vi "诊断标定3 - 副本.vi"(8 "CAN端口":u16(ring), 9 "设备索引号":u16(ring), 10 "CAN卡类型":u32(ring)=21) -> ()   [LabVIEW 2013] (continued)
            n1286 = Select(t=0, s=w1771, f=1) -> (s? t:f=w1770:i32)
            n1287 = property on="电池实际容量(A)" class="DigNum (严格)"("Disabled"=w1770) -> ()  [unwired: 2 in, 2 out]
            n1288 = property on="电池额定容量(A)" class="DigNum (严格)"("Disabled"=w1770) -> ()  [unwired: 2 in, 2 out]
            n1289 = property on="项目信息2" class="Clust (严格)"("DisabledEnum"=w1770) -> ()  [unwired: 2 in, 2 out]
            n1290 = global read "功能码全局.vi" "主板项目信息7"() -> (w1777:bool[])
            n1291 = Index Array(array=w1777, index #1=3 ("索引"), index #2=6 ("索引")) -> (element #1=w1775:bool, element #2=w1774:bool)
            n1292 = Not(x=w1781) -> (.not. x?=w1780:bool)
          }
          frame "配置文件版本" {
            w1794 = 2
            w1796 = FALSE
            n1293 = property on="使用者" class="DigNum (严格)"("Disabled"=w1794) -> ()  [unwired: 2 in, 2 out]
            n1294 = property on="SOH(%)" class="DigNum (严格)"("Disabled"=w1794) -> ()  [unwired: 2 in, 2 out]
            n1295 = property on="SOC(%)" class="DigNum (严格)"("Disabled"=w1794) -> ()  [unwired: 2 in, 2 out]
            n1296 = property on="电池实际容量(A)" class="DigNum (严格)"("Disabled"=w1794) -> ()  [unwired: 2 in, 2 out]
            n1297 = property on="从板个数" class="DigNum (严格)"("NumText.BGColor"=u32 13816530) -> ()  [unwired: 2 in, 2 out]
            n1298 = property on="电池额定容量(A)" class="DigNum (严格)"("Disabled"=w1794) -> ()  [unwired: 2 in, 2 out]
            n1299 = property on="系统时钟" class="Str"("Disabled"=w1794) -> ()  [unwired: 2 in, 2 out]
            n1300 = property on="车架(牌)号" class="Str"("Disabled"=w1794) -> ()  [unwired: 2 in, 2 out]
            n1301 = property on="项目信息" class="Tbl (严格)"("Disabled"=w1794) -> ()  [unwired: 2 in, 2 out]
            n1302 = property on="产品编号" class="Str"("Disabled"=w1794) -> ()  [unwired: 2 in, 2 out]
            n1303 = Select(t=0, s=w1785, f=1) -> (s? t:f=w1784:i32)
            n1304 = property on="项目信息2" class="Clust (严格)"("DisabledEnum"=w1784) -> ()  [unwired: 2 in, 2 out]
            n1305 = property on="配置文件版本" class="Str"("Disabled"=w1784) -> ()  [unwired: 2 in, 2 out]
            n1306 = global read "功能码全局.vi" "主板项目信息5"() -> (w1792:bool[])
            n1307 = global read "功能码全局.vi" "主板项目信息6"() -> (w1791:bool[])
            n1308 = Index Array(array=w1792, index=6 ("索引")) -> (element=w1789:bool)
            n1309 = Index Array(array=w1791, index=7 ("索引")) -> (element=w1788:bool)
            n1310 = Not(x=w1796) -> (.not. x?=w1795:bool)
          }
          frame "参数修改记录" {
            w1809 = 2
            w1811 = FALSE
            n1311 = property on="SOH(%)" class="DigNum (严格)"("Disabled"=w1809) -> ()  [unwired: 2 in, 2 out]
            n1312 = property on="SOC(%)" class="DigNum (严格)"("Disabled"=w1809) -> ()  [unwired: 2 in, 2 out]
            n1313 = property on="电池实际容量(A)" class="DigNum (严格)"("Disabled"=w1809) -> ()  [unwired: 2 in, 2 out]
            n1314 = property on="电池额定容量(A)" class="DigNum (严格)"("Disabled"=w1809) -> ()  [unwired: 2 in, 2 out]
            n1315 = property on="从板个数" class="DigNum (严格)"("NumText.BGColor"=u32 13816530) -> ()  [unwired: 2 in, 2 out]
            n1316 = property on="系统时钟" class="Str"("Disabled"=w1809) -> ()  [unwired: 2 in, 2 out]
            n1317 = property on="车架(牌)号" class="Str"("Disabled"=w1809) -> ()  [unwired: 2 in, 2 out]
            n1318 = property on="配置文件版本" class="Str"("Disabled"=w1809) -> ()  [unwired: 2 in, 2 out]
            n1319 = property on="项目信息" class="Tbl (严格)"("Disabled"=w1809) -> ()  [unwired: 2 in, 2 out]
            n1320 = property on="产品编号" class="Str"("Disabled"=w1809) -> ()  [unwired: 2 in, 2 out]
            n1321 = Select(t=0, s=w1800, f=1) -> (s? t:f=w1799:i32)
            n1322 = property on="使用者" class="DigNum (严格)"("Disabled"=w1799) -> ()  [unwired: 2 in, 2 out]
            n1323 = property on="项目信息2" class="Clust (严格)"("DisabledEnum"=w1799) -> ()  [unwired: 2 in, 2 out]
            n1324 = global read "功能码全局.vi" "主板项目信息7"() -> (w1806:bool[])
            n1325 = global read "功能码全局.vi" "主板项目信息5"() -> (w1807:bool[])
            n1326 = Index Array(array=w1806, index=0 ("索引")) -> (element=w1804:bool)
            n1327 = Index Array(array=w1807, index=7 ("索引")) -> (element=w1803:bool)
            n1328 = Not(x=w1811) -> (.not. x?=w1810:bool)
          }
          frame "车牌号" {
            w1824 = 2
            w1826 = FALSE
            n1329 = property on="SOH(%)" class="DigNum (严格)"("Disabled"=w1824) -> ()  [unwired: 2 in, 2 out]
            n1330 = property on="使用者" class="DigNum (严格)"("Disabled"=w1824) -> ()  [unwired: 2 in, 2 out]
            n1331 = property on="SOC(%)" class="DigNum (严格)"("Disabled"=w1824) -> ()  [unwired: 2 in, 2 out]
            n1332 = property on="电池实际容量(A)" class="DigNum (严格)"("Disabled"=w1824) -> ()  [unwired: 2 in, 2 out]
            n1333 = property on="电池额定容量(A)" class="DigNum (严格)"("Disabled"=w1824) -> ()  [unwired: 2 in, 2 out]
            n1334 = property on="从板个数" class="DigNum (严格)"("NumText.BGColor"=u32 13816530) -> ()  [unwired: 2 in, 2 out]
            n1335 = property on="系统时钟" class="Str"("Disabled"=w1824) -> ()  [unwired: 2 in, 2 out]
            n1336 = property on="配置文件版本" class="Str"("Disabled"=w1824) -> ()  [unwired: 2 in, 2 out]
            n1337 = property on="项目信息" class="Tbl (严格)"("Disabled"=w1824) -> ()  [unwired: 2 in, 2 out]
            n1338 = property on="产品编号" class="Str"("Disabled"=w1824) -> ()  [unwired: 2 in, 2 out]
            n1339 = Select(t=0, s=w1815, f=1) -> (s? t:f=w1814:i32)
            n1340 = property on="车架(牌)号" class="Str"("Disabled"=w1814) -> ()  [unwired: 2 in, 2 out]
            n1341 = property on="项目信息2" class="Clust (严格)"("DisabledEnum"=w1814) -> ()  [unwired: 2 in, 2 out]
            n1342 = global read "功能码全局.vi" "主板项目信息7"() -> (w1821:bool[])
            n1343 = global read "功能码全局.vi" "主板项目信息6"() -> (w1822:bool[])
            n1344 = Index Array(array=w1821, index=1 ("索引")) -> (element=w1819:bool)
            n1345 = Index Array(array=w1822, index=0 ("索引")) -> (element=w1818:bool)
            n1346 = Not(x=w1826) -> (.not. x?=w1825:bool)
          }
          frame "SOH" {
            w1838 = 2
            w1840 = FALSE
            n1347 = property on="使用者" class="DigNum (严格)"("Disabled"=w1838) -> ()  [unwired: 2 in, 2 out]
            n1348 = property on="SOC(%)" class="DigNum (严格)"("Disabled"=w1838) -> ()  [unwired: 2 in, 2 out]
            n1349 = property on="电池实际容量(A)" class="DigNum (严格)"("Disabled"=w1838) -> ()  [unwired: 2 in, 2 out]
            n1350 = property on="电池额定容量(A)" class="DigNum (严格)"("Disabled"=w1838) -> ()  [unwired: 2 in, 2 out]
            n1351 = property on="从板个数" class="DigNum (严格)"("NumText.BGColor"=u32 13816530) -> ()  [unwired: 2 in, 2 out]
            n1352 = property on="系统时钟" class="Str"("Disabled"=w1838) -> ()  [unwired: 2 in, 2 out]
            n1353 = property on="配置文件版本" class="Str"("Disabled"=w1838) -> ()  [unwired: 2 in, 2 out]
            n1354 = property on="项目信息" class="Tbl (严格)"("Disabled"=w1838) -> ()  [unwired: 2 in, 2 out]
            n1355 = property on="产品编号" class="Str"("Disabled"=w1838) -> ()  [unwired: 2 in, 2 out]
            n1356 = property on="车架(牌)号" class="Str"("Disabled"=w1838) -> ()  [unwired: 2 in, 2 out]
            n1357 = Select(t=0, s=w1830, f=1) -> (s? t:f=w1829:i32)
            n1358 = property on="项目信息2" class="Clust (严格)"("DisabledEnum"=w1829) -> ()  [unwired: 2 in, 2 out]
            n1359 = property on="SOH(%)" class="DigNum (严格)"("Disabled"=w1829) -> ()  [unwired: 2 in, 2 out]
            n1360 = global read "功能码全局.vi" "主板项目信息7"() -> (w1837:bool[])
            n1361 = Index Array(array=w1837, index #1=4 ("索引"), index #2=7 ("索引")) -> (element #1=w1834:bool, element #2=w1833:bool)
            n1362 = Not(x=w1840) -> (.not. x?=w1839:bool)
          }
          frame "SOC过低(2)", "SOC过高(2)", "SOH过低(2)", "充电电流过高(2)", "单体电压过低(2)", "单体电压过高(2)", "单组电压不均衡(2)", "单组温度不均衡(2)", "二级故障阀值", "放电电流过高(2)", "极柱温度过高(2)", "内阻过大(2)", "温度过低(2)", "温度过高(2)", "整组电压不均衡(2)", "整组温度不均衡(2)", "总电压过低(2)", "总电压过高(2)" {
            w1852 = FALSE
            n1363 = property on="从板个数" class="DigNum (严格)"("NumText.BGColor"=u32 13816530) -> ()  [unwired: 2 in, 2 out]
            n1364 = Select(t=0, s=w1844, f=1) -> (s? t:f=w1843:i32)
            n1365 = property on="一级故障 2" class="Clust (严格)"("DisabledEnum"=w1843) -> ()  [unwired: 2 in, 2 out]
            n1366 = global read "功能码全局.vi" "主板故障阀值9"() -> (w1850:bool[])
            n1367 = Index Array(array=w1850, index #1=3 ("索引"), index #2=6 ("索引")) -> (element #1=w1848:bool, element #2=w1847:bool)
            n1368 = Not(x=w1852) -> (.not. x?=w1853:bool)
          }
          frame "SOC过低(3)", "SOC过高(3)", "SOH过低(3)", "充电电流过高(3)", "单体电压过低(3)", "单体电压过高(3)", "单组电压不均衡(3)", "单组温度不均衡(3)", "放电电流过高(3)", "极柱温度过高(3)", "内阻过大(3)", "三级故障阀值", "温度过低(3)", "温度过高(3)", "整组电压不均衡(3)", "整组温度不均衡(3)", "总电压过低(3)", "总电压过高(3)" {
            w1866 = FALSE
            n1369 = property on="从板个数" class="DigNum (严格)"("NumText.BGColor"=u32 13816530) -> ()  [unwired: 2 in, 2 out]
            n1370 = Select(t=0, s=w1857, f=1) -> (s? t:f=w1856:i32)
            n1371 = property on="一级故障 3" class="Clust (严格)"("DisabledEnum"=w1856) -> ()  [unwired: 2 in, 2 out]
            n1372 = global read "功能码全局.vi" "主板故障阀值9"() -> (w1863:bool[])
            n1373 = Index Array(array=w1863, index #1=4 ("索引"), index #2=7 ("索引")) -> (element #1=w1861:bool, element #2=w1860:bool)
            n1374 = Not(x=w1866) -> (.not. x?=w1865:bool)
          }
          frame "SOC过低", "SOC过高", "SOH过低", "充电电流过高", "单体电压过低", "单体电压过高", "单组电压不均衡", "单组温度不均衡", "放电电流过高", "极柱温度过高", "内阻过大", "温度过低", "温度过高", "一级故障阀值", "整组电压不均衡", "整组温度不均衡", "总电压过低", "总电压过高" {
            w1879 = FALSE
            n1375 = Select(t=0, s=w1870, f=1) -> (s? t:f=w1869:i32)
            n1376 = property on="从板个数" class="DigNum (严格)"("NumText.BGColor"=u32 13816530) -> ()  [unwired: 2 in, 2 out]
            n1377 = property on="一级故障" class="Clust (严格)"("DisabledEnum"=w1869) -> ()  [unwired: 2 in, 2 out]
            n1378 = global read "功能码全局.vi" "主板故障阀值9"() -> (w1876:bool[])
            n1379 = Index Array(array=w1876, index #1=2 ("索引"), index #2=5 ("索引")) -> (element #1=w1874:bool, element #2=w1873:bool)
            n1380 = Not(x=w1879) -> (.not. x?=w1878:bool)
          }
          frame "充电控制参数", "电流步长", "最大允许充电电流", "最大允许充电温度", "最大允许单体电压", "最大允许总电压", "最小允许充电电流", "最小允许充电温度", "最小允许单体电压" {
            w1882 = 2
            w1893 = FALSE
            n1381 = property on="从板个数" class="DigNum (严格)"("NumText.BGColor"=u32 13816530) -> ()  [unwired: 2 in, 2 out]
            n1382 = property on="风机开启温度" class="DigNum (严格)"("Disabled"=w1882) -> ()  [unwired: 2 in, 2 out]
            n1383 = property on="风机关闭温度" class="DigNum (严格)"("Disabled"=w1882) -> ()  [unwired: 2 in, 2 out]
            n1384 = property on="加热开启温度" class="DigNum (严格)"("Disabled"=w1882) -> ()  [unwired: 2 in, 2 out]
            n1385 = property on="加热关闭温度" class="DigNum (严格)"("Disabled"=w1882) -> ()  [unwired: 2 in, 2 out]
            n1386 = property on="风机开启温差" class="DigNum (严格)"("Disabled"=w1882) -> ()  [unwired: 2 in, 2 out]
            n1387 = property on="风机关闭温差" class="DigNum (严格)"("Disabled"=w1882) -> ()  [unwired: 2 in, 2 out]
            n1388 = property on="加热控制参数" class="Clust (严格)"("DisabledEnum"=w1882) -> ()  [unwired: 2 in, 2 out]
            n1389 = Select(t=0, s=w1884, f=1) -> (s? t:f=w1883:i32)
            n1390 = property on="最大允许总电压" class="DigNum (严格)"("Disabled"=w1883) -> ()  [unwired: 2 in, 2 out]
            n1391 = property on="最大允许充电温度" class="DigNum (严格)"("Disabled"=w1883) -> ()  [unwired: 2 in, 2 out]
            n1392 = property on="最小允许充电温度" class="DigNum (严格)"("Disabled"=w1883) -> ()  [unwired: 2 in, 2 out]
            n1393 = property on="电流步长" class="DigNum (严格)"("Disabled"=w1883) -> ()  [unwired: 2 in, 2 out]
            n1394 = property on="最大允许单体电压" class="DigNum (严格)"("Disabled"=w1883) -> ()  [unwired: 2 in, 2 out]
            n1395 = property on="最小允许单体电压" class="DigNum (严格)"("Disabled"=w1883) -> ()  [unwired: 2 in, 2 out]
            n1396 = property on="最大允许充电电流" class="DigNum (严格)"("Disabled"=w1883) -> ()  [unwired: 2 in, 2 out]
            n1397 = property on="最小允许充电电流" class="DigNum (严格)"("Disabled"=w1883) -> ()  [unwired: 2 in, 2 out]
            n1398 = global read "功能码全局.vi" "主板控制类信息10"() -> (w1890:bool[])
            n1399 = Index Array(array=w1890, index #1=5 ("索引"), index #2=7 ("索引")) -> (element #1=w1888:bool, element #2=w1887:bool)
            n1400 = Not(x=w1893) -> (.not. x?=w1892:bool)
          }
          frame "风机关闭温差", "风机关闭温度", "风机开启温差", "风机开启温度", "加热关闭温差", "加热关闭温度", "加热开启温度", "加热控制参数" {
            w1905 = 2
            w1907 = FALSE
            n1401 = Select(t=0, s=w1897, f=1) -> (s? t:f=w1896:i32)
            n1402 = property on="从板个数" class="DigNum (严格)"("NumText.BGColor"=u32 13816530) -> ()  [unwired: 2 in, 2 out]
            n1403 = property on="加热控制参数" class="Clust (严格)"("DisabledEnum"=w1896) -> ()  [unwired: 2 in, 2 out]
            n1404 = property on="风机开启温度" class="DigNum (严格)"("Disabled"=w1896) -> ()  [unwired: 2 in, 2 out]
            n1405 = property on="风机关闭温度" class="DigNum (严格)"("Disabled"=w1896) -> ()  [unwired: 2 in, 2 out]
            n1406 = property on="加热开启温度" class="DigNum (严格)"("Disabled"=w1896) -> ()  [unwired: 2 in, 2 out]
            n1407 = property on="加热关闭温度" class="DigNum (严格)"("Disabled"=w1896) -> ()  [unwired: 2 in, 2 out]
            n1408 = property on="风机开启温差" class="DigNum (严格)"("Disabled"=w1896) -> ()  [unwired: 2 in, 2 out]
            n1409 = property on="风机关闭温差" class="DigNum (严格)"("Disabled"=w1896) -> ()  [unwired: 2 in, 2 out]
            n1410 = property on="最大允许总电压" class="DigNum (严格)"("Disabled"=w1905) -> ()  [unwired: 2 in, 2 out]
            n1411 = property on="最大允许充电温度" class="DigNum (严格)"("Disabled"=w1905) -> ()  [unwired: 2 in, 2 out]
            n1412 = property on="最小允许充电温度" class="DigNum (严格)"("Disabled"=w1905) -> ()  [unwired: 2 in, 2 out]
            n1413 = property on="电流步长" class="DigNum (严格)"("Disabled"=w1905) -> ()  [unwired: 2 in, 2 out]
            n1414 = property on="最大允许单体电压" class="DigNum (严格)"("Disabled"=w1905) -> ()  [unwired: 2 in, 2 out]
            n1415 = property on="最小允许单体电压" class="DigNum (严格)"("Disabled"=w1905) -> ()  [unwired: 2 in, 2 out]
            n1416 = property on="最大允许充电电流" class="DigNum (严格)"("Disabled"=w1905) -> ()  [unwired: 2 in, 2 out]
            n1417 = property on="最小允许充电电流" class="DigNum (严格)"("Disabled"=w1905) -> ()  [unwired: 2 in, 2 out]
            n1418 = global read "功能码全局.vi" "主板控制类信息10"() -> (w1903:bool[])
            n1419 = Index Array(array=w1903, index #1=4 ("索引"), index #2=6 ("索引")) -> (element #1=w1901:bool, element #2=w1900:bool)
            n1420 = Not(x=w1907) -> (.not. x?=w1906:bool)
          }
          frame "电池信息" {
            w1920 = FALSE
            n1421 = Select(t=0, s=w1911, f=1) -> (s? t:f=w1910:i32)
            n1422 = property on="电池串联" class="DigNum (严格)"("Disabled"=w1910) -> ()  [unwired: 2 in, 2 out]
            n1423 = property on="电池并联" class="DigNum (严格)"("Disabled"=w1910) -> ()  [unwired: 2 in, 2 out]
            n1424 = property on="电池包额定容量" class="DigNum (严格)"("Disabled"=w1910) -> ()  [unwired: 2 in, 2 out]
            n1425 = property on="电池包额定能量(kWh)" class="DigNum (严格)"("Disabled"=w1910) -> ()  [unwired: 2 in, 2 out]
            n1426 = property on="电池包额定总电压" class="DigNum (严格)"("Disabled"=w1910) -> ()  [unwired: 2 in, 2 out]
            n1427 = property on="实际容量" class="DigNum (严格)"("Disabled"=w1910) -> ()  [unwired: 2 in, 2 out]
            n1428 = property on="电池包组号" class="Str"("Disabled"=w1910) -> ()  [unwired: 2 in, 2 out]
            n1429 = property on="电池生产日期" class="Str"("Disabled"=w1910) -> ()  [unwired: 2 in, 2 out]
            n1430 = property on="电池厂家" class="Str"("Disabled"=w1910) -> ()  [unwired: 2 in, 2 out]
            n1431 = property on="电池类型" class="Str"("Disabled"=w1910) -> ()  [unwired: 2 in, 2 out]
            n1432 = property on="累计充电总安时" class="DigNum (严格)"("Disabled"=w1910) -> ()  [unwired: 2 in, 2 out]
            n1433 = property on="累计放电总安时" class="DigNum (严格)"("Disabled"=w1910) -> ()  [unwired: 2 in, 2 out]
            n1434 = property on="电池放空次数" class="DigNum (严格)"("Disabled"=w1910) -> ()  [unwired: 2 in, 2 out]
            n1435 = property on="电池充满次数" class="DigNum (严格)"("Disabled"=w1910) -> ()  [unwired: 2 in, 2 out]
            n1436 = property on="电池充电次数" class="DigNum (严格)"("Disabled"=w1910) -> ()  [unwired: 2 in, 2 out]
            n1437 = property on="电池信息" class="Clust (严格)"("DisabledEnum"=w1910) -> ()  [unwired: 2 in, 2 out]
            n1438 = global read "功能码全局.vi" "主板版本号11"() -> (w1917:bool[])
            n1439 = property on="从板个数" class="DigNum (严格)"("NumText.BGColor"=u32 13816530) -> ()  [unwired: 2 in, 2 out]
            n1440 = Index Array(array=w1917, index #1=0 ("索引"), index #2=1 ("索引")) -> (element #1=w1915:bool, element #2=w1914:bool)
            n1441 = Not(x=w1920) -> (.not. x?=w1919:bool)
          }
          frame "电池信息1" {
            w1932 = 2
            w1934 = FALSE
            n1442 = Select(t=0, s=w1924, f=1) -> (s? t:f=w1923:i32)
            n1443 = property on="电池信息" class="Clust (严格)"("DisabledEnum"=w1923) -> ()  [unwired: 2 in, 2 out]
            n1444 = property on="电池生产日期" class="Str"("Disabled"=w1923) -> ()  [unwired: 2 in, 2 out]
            n1445 = property on="电池厂家" class="Str"("Disabled"=w1923) -> ()  [unwired: 2 in, 2 out]
            n1446 = property on="电池类型" class="Str"("Disabled"=w1923) -> ()  [unwired: 2 in, 2 out]
            n1447 = property on="电池串联" class="DigNum (严格)"("Disabled"=w1923) -> ()  [unwired: 2 in, 2 out]
            n1448 = property on="电池并联" class="DigNum (严格)"("Disabled"=w1923) -> ()  [unwired: 2 in, 2 out]
            n1449 = property on="电池包额定容量" class="DigNum (严格)"("Disabled"=w1923) -> ()  [unwired: 2 in, 2 out]
            n1450 = property on="电池包额定能量(kWh)" class="DigNum (严格)"("Disabled"=w1923) -> ()  [unwired: 2 in, 2 out]
            n1451 = property on="电池包额定总电压" class="DigNum (严格)"("Disabled"=w1923) -> ()  [unwired: 2 in, 2 out]
            n1452 = property on="实际容量" class="DigNum (严格)"("Disabled"=w1923) -> ()  [unwired: 2 in, 2 out]
            n1453 = property on="累计充电总安时" class="DigNum (严格)"("Disabled"=w1932) -> ()  [unwired: 2 in, 2 out]
            n1454 = property on="累计放电总安时" class="DigNum (严格)"("Disabled"=w1932) -> ()  [unwired: 2 in, 2 out]
            n1455 = property on="电池放空次数" class="DigNum (严格)"("Disabled"=w1932) -> ()  [unwired: 2 in, 2 out]
            n1456 = property on="电池充满次数" class="DigNum (严格)"("Disabled"=w1932) -> ()  [unwired: 2 in, 2 out]
            n1457 = property on="电池充电次数" class="DigNum (严格)"("Disabled"=w1932) -> ()  [unwired: 2 in, 2 out]
            n1458 = property on="从板个数" class="DigNum (严格)"("NumText.BGColor"=u32 13816530) -> ()  [unwired: 2 in, 2 out]
            n1459 = property on="电池包组号" class="Str"("Disabled"=w1932) -> ()  [unwired: 2 in, 2 out]
            n1460 = global read "功能码全局.vi" "主板版本号11"() -> (w1930:bool[])
            n1461 = Index Array(array=w1930, index #1=0 ("索引"), index #2=1 ("索引")) -> (element #1=w1928:bool, element #2=w1927:bool)
            n1462 = Not(x=w1934) -> (.not. x?=w1933:bool)
          }
          frame "电池包组号" {
            w1946 = 2
            w1948 = FALSE
            n1463 = property on="电池生产日期" class="Str"("Disabled"=w1946) -> ()  [unwired: 2 in, 2 out]
            n1464 = property on="电池厂家" class="Str"("Disabled"=w1946) -> ()  [unwired: 2 in, 2 out]
            n1465 = property on="电池类型" class="Str"("Disabled"=w1946) -> ()  [unwired: 2 in, 2 out]
            n1466 = property on="电池串联" class="DigNum (严格)"("Disabled"=w1946) -> ()  [unwired: 2 in, 2 out]
            n1467 = property on="电池并联" class="DigNum (严格)"("Disabled"=w1946) -> ()  [unwired: 2 in, 2 out]
            n1468 = property on="电池包额定容量" class="DigNum (严格)"("Disabled"=w1946) -> ()  [unwired: 2 in, 2 out]
            n1469 = property on="电池包额定能量(kWh)" class="DigNum (严格)"("Disabled"=w1946) -> ()  [unwired: 2 in, 2 out]
            n1470 = property on="电池包额定总电压" class="DigNum (严格)"("Disabled"=w1946) -> ()  [unwired: 2 in, 2 out]
            n1471 = property on="实际容量" class="DigNum (严格)"("Disabled"=w1946) -> ()  [unwired: 2 in, 2 out]
            n1472 = property on="从板个数" class="DigNum (严格)"("NumText.BGColor"=u32 13816530) -> ()  [unwired: 2 in, 2 out]
            n1473 = property on="累计充电总安时" class="DigNum (严格)"("Disabled"=w1946) -> ()  [unwired: 2 in, 2 out]
            n1474 = property on="累计放电总安时" class="DigNum (严格)"("Disabled"=w1946) -> ()  [unwired: 2 in, 2 out]
            n1475 = property on="电池放空次数" class="DigNum (严格)"("Disabled"=w1946) -> ()  [unwired: 2 in, 2 out]
            n1476 = property on="电池充满次数" class="DigNum (严格)"("Disabled"=w1946) -> ()  [unwired: 2 in, 2 out]
            n1477 = property on="电池充电次数" class="DigNum (严格)"("Disabled"=w1946) -> ()  [unwired: 2 in, 2 out]
            n1478 = Select(t=0, s=w1938, f=1) -> (s? t:f=w1937:i32)
            n1479 = property on="电池包组号" class="Str"("Disabled"=w1937) -> ()  [unwired: 2 in, 2 out]
            n1480 = property on="电池信息" class="Clust (严格)"("DisabledEnum"=w1937) -> ()  [unwired: 2 in, 2 out]
            n1481 = global read "功能码全局.vi" "主板版本号11"() -> (w1944:bool[])
            n1482 = Index Array(array=w1944, index #1=0 ("索引"), index #2=1 ("索引")) -> (element #1=w1942:bool, element #2=w1941:bool)
            n1483 = Not(x=w1948) -> (.not. x?=w1947:bool)
          }
          frame "充放电安时" {
            w1960 = 2
            w1962 = FALSE
            n1484 = property on="电池生产日期" class="Str"("Disabled"=w1960) -> ()  [unwired: 2 in, 2 out]
            n1485 = property on="电池厂家" class="Str"("Disabled"=w1960) -> ()  [unwired: 2 in, 2 out]
            n1486 = property on="电池类型" class="Str"("Disabled"=w1960) -> ()  [unwired: 2 in, 2 out]
            n1487 = property on="电池串联" class="DigNum (严格)"("Disabled"=w1960) -> ()  [unwired: 2 in, 2 out]
            n1488 = property on="电池并联" class="DigNum (严格)"("Disabled"=w1960) -> ()  [unwired: 2 in, 2 out]
            n1489 = property on="电池包额定容量" class="DigNum (严格)"("Disabled"=w1960) -> ()  [unwired: 2 in, 2 out]
            n1490 = property on="电池包额定能量(kWh)" class="DigNum (严格)"("Disabled"=w1960) -> ()  [unwired: 2 in, 2 out]
            n1491 = property on="电池包额定总电压" class="DigNum (严格)"("Disabled"=w1960) -> ()  [unwired: 2 in, 2 out]
            n1492 = property on="实际容量" class="DigNum (严格)"("Disabled"=w1960) -> ()  [unwired: 2 in, 2 out]
            n1493 = property on="从板个数" class="DigNum (严格)"("NumText.BGColor"=u32 13816530) -> ()  [unwired: 2 in, 2 out]
            n1494 = Select(t=0, s=w1952, f=1) -> (s? t:f=w1951:i32)
            n1495 = property on="电池放空次数" class="DigNum (严格)"("Disabled"=w1960) -> ()  [unwired: 2 in, 2 out]
            n1496 = property on="电池充满次数" class="DigNum (严格)"("Disabled"=w1960) -> ()  [unwired: 2 in, 2 out]
            n1497 = property on="电池充电次数" class="DigNum (严格)"("Disabled"=w1960) -> ()  [unwired: 2 in, 2 out]
            n1498 = property on="电池包组号" class="Str"("Disabled"=w1960) -> ()  [unwired: 2 in, 2 out]
            n1499 = property on="累计充电总安时" class="DigNum (严格)"("Disabled"=w1951) -> ()  [unwired: 2 in, 2 out]
            n1500 = property on="累计放电总安时" class="DigNum (严格)"("Disabled"=w1951) -> ()  [unwired: 2 in, 2 out]
            n1501 = property on="电池信息" class="Clust (严格)"("DisabledEnum"=w1951) -> ()  [unwired: 2 in, 2 out]
            n1502 = global read "功能码全局.vi" "主板版本号11"() -> (w1958:bool[])
            n1503 = Index Array(array=w1958, index #1=0 ("索引"), index #2=1 ("索引")) -> (element #1=w1956:bool, element #2=w1955:bool)
            n1504 = Not(x=w1962) -> (.not. x?=w1961:bool)
          }
          frame "电池充放电次数" {
            w1974 = 2
            w1976 = FALSE
            n1505 = property on="从板个数" class="DigNum (严格)"("NumText.BGColor"=u32 13816530) -> ()  [unwired: 2 in, 2 out]
            n1506 = property on="电池生产日期" class="Str"("Disabled"=w1974) -> ()  [unwired: 2 in, 2 out]
            n1507 = property on="电池厂家" class="Str"("Disabled"=w1974) -> ()  [unwired: 2 in, 2 out]
            n1508 = property on="电池类型" class="Str"("Disabled"=w1974) -> ()  [unwired: 2 in, 2 out]
            n1509 = property on="电池串联" class="DigNum (严格)"("Disabled"=w1974) -> ()  [unwired: 2 in, 2 out]
            n1510 = property on="电池并联" class="DigNum (严格)"("Disabled"=w1974) -> ()  [unwired: 2 in, 2 out]
            n1511 = property on="电池包额定容量" class="DigNum (严格)"("Disabled"=w1974) -> ()  [unwired: 2 in, 2 out]
            n1512 = property on="电池包额定能量(kWh)" class="DigNum (严格)"("Disabled"=w1974) -> ()  [unwired: 2 in, 2 out]
            n1513 = property on="电池包额定总电压" class="DigNum (严格)"("Disabled"=w1974) -> ()  [unwired: 2 in, 2 out]
            n1514 = property on="实际容量" class="DigNum (严格)"("Disabled"=w1974) -> ()  [unwired: 2 in, 2 out]
            n1515 = Select(t=0, s=w1966, f=1) -> (s? t:f=w1965:i32)
            n1516 = property on="电池放空次数" class="DigNum (严格)"("Disabled"=w1965) -> ()  [unwired: 2 in, 2 out]
            n1517 = property on="电池充满次数" class="DigNum (严格)"("Disabled"=w1965) -> ()  [unwired: 2 in, 2 out]
            n1518 = property on="电池充电次数" class="DigNum (严格)"("Disabled"=w1965) -> ()  [unwired: 2 in, 2 out]
            n1519 = property on="累计充电总安时" class="DigNum (严格)"("Disabled"=w1974) -> ()  [unwired: 2 in, 2 out]
            n1520 = property on="累计放电总安时" class="DigNum (严格)"("Disabled"=w1974) -> ()  [unwired: 2 in, 2 out]
            n1521 = property on="电池信息" class="Clust (严格)"("DisabledEnum"=w1965) -> ()  [unwired: 2 in, 2 out]
            n1522 = property on="电池包组号" class="Str"("Disabled"=w1974) -> ()  [unwired: 2 in, 2 out]
            n1523 = global read "功能码全局.vi" "主板版本号11"() -> (w1972:bool[])
            n1524 = Index Array(array=w1972, index #1=0 ("索引"), index #2=1 ("索引")) -> (element #1=w1970:bool, element #2=w1969:bool)
            n1525 = Not(x=w1976) -> (.not. x?=w1975:bool)
          }
          frame "假", Default {
            w1981 = FALSE
            n1526 = Not(x=w1981) -> (.not. x?=w1980:bool)
          }
        }
        n1527 = property on="单个读取" class="Bool (严格)"("Visible"=w1449) -> ()  [unwired: 2 in, 2 out]
        n1528 = property on="单个写入" class="Bool (严格)"("Visible"=w1448) -> ()  [unwired: 2 in, 2 out]
        n1529 = local write "1"(w1456) -> ()
        n1530 = local write "1 2"(w1455) -> ()
        n1531 = local write "1 3"(w1454) -> ()
        n1532 = local write "1 4"(w1453) -> ()
        n1533 = local write "1 5"(w1452) -> ()
        n1534 = local write "1 11"(w1451) -> ()
        n1535 = local write "主板2"(w1457) -> ()
      }
      event "从板选项": Mouse Down {
        n1536 = event-data() -> ("CtlRef"=w1996:refnum<vi>)  [unwired: 8 out]
        n1537 = property class="Tree (严格)"(reference=w1996) -> ("Value"=w1995:string)  [unwired: 1 in, 2 out]
        n1538 = global read "功能码全局.vi" "主板监控2"() -> (w1986:bool[])
        n1539 = Index Array(array=w1986, index=6 ("索引")) -> (element=w1984:bool)
        n1540 = case shown="\"二维码\"" w1995 {
          tunnel: [T19."从板信息" ("等级 2") T19."从板信息" ("等级 2") T19."从板信息" ("等级 2") T19."从板信息" ("等级 2") T19."从板信息" ("等级 2") T19."从板信息" ("等级 2") T19."从板信息" ("等级 2") T19."从板信息" ("等级 2") T19."一级故障阀值" ("等级 2") T19."二级故障阀值" ("等级 2") T19."三级故障阀值" ("等级 2") T19."快换参数" ("等级 2") T19."快换参数" ("等级 2") T19."快换参数" ("等级 2") T19."快换参数" ("等级 2") T19."快换参数" ("等级 2") T19."快换参数" ("等级 2") T19."快换参数" ("等级 2") T19."快换参数" ("等级 2") T14."均衡参数" ("等级 2") T14."均衡参数" ("等级 2") T14."均衡参数" ("等级 2") T19."从板信息" ("等级 2")] -> w1994
          tunnel: [w2007 w2017 w2027 w2041 w2056 w2091 w2128 w2165 w2189 w2202 w2215 w2228 w2254 w2268 w2284 w2301 w2318 w2336 w2355 w2372 w2385 w2399 w2414] -> w1993
          tunnel: [w1999 w2009 w2019 w2029 w2043 w2078 w2115 w2152 w2200 w2202 w2215 w2228 w2254 w2268 w2284 w2301 w2318 w2336 w2355 w2372 w2385 w2399 w2413] -> w1992
          tunnel: [w1999 w2009 w2019 w2029 w2043 w2078 w2115 w2152 w2189 w2213 w2215 w2228 w2254 w2268 w2284 w2301 w2318 w2336 w2355 w2372 w2385 w2399 w2413] -> w1991
          tunnel: [w1999 w2009 w2019 w2029 w2043 w2078 w2115 w2152 w2189 w2202 w2226 w2228 w2254 w2268 w2284 w2301 w2318 w2336 w2355 w2372 w2385 w2399 w2413] -> w1990
          tunnel: [w1999 w2009 w2019 w2029 w2043 w2078 w2115 w2152 w2189 w2202 w2215 w2252 w2266 w2282 w2299 w2316 w2334 w2353 w2370 w2372 w2385 w2399 w2413] -> w1989
          tunnel: [w2004 w2014 w2020 w2036 w2050 w2085 w2122 w2159 w2196 w2209 w2222 w2237 w2259 w2274 w2288 w2306 w2321 w2341 w2359 w2375 w2389 w2404 w2413] -> w1988
          tunnel: [w2001 w2011 w2020 w2035 w2049 w2084 w2121 w2158 w2195 w2208 w2221 w2229 w2258 w2273 w2287 w2307 w2322 w2340 w2358 w2374 w2388 w2403 w2413] -> w1987
          tunnel: w1984 -> [_ _ w2024 w2032 w2046 w2081 w2118 w2155 w2191 w2205 w2218 w2249 w2262 w2277 w2292 w2310 w2326 w2344 w2363 w2378 w2392 w2406 _]
          tunnel: [w1999 w2009 w2019 w2029 w2043 w2078 w2115 w2152 w2189 w2202 w2215 w2228 w2254 w2268 w2284 w2301 w2318 w2336 w2355 w2373 w2386 w2400 w2413] -> w1983
          frame "从板号" {
            w2006 = 2
            w1999 = FALSE ("1 6")
            n1541 = property on="项目信息 2" class="Tbl (严格)"("Disabled"=w2006) -> ()  [unwired: 2 in, 2 out]
            n1542 = property on="加热控制参数" class="Clust (严格)"("Disabled"=w2006) -> ()  [unwired: 2 in, 2 out]
            n1543 = property on="从板号" class="DigNum (严格)"("NumText.BGColor"=u32 6618880) -> ()  [unwired: 2 in, 2 out]
            n1544 = global read "功能码全局.vi" "16"() -> (w2003:bool[])
            n1545 = Index Array(array=w2003, index #1=4 ("索引"), index #2=6 ("索引")) -> (element #1=w2004:bool, element #2=w2001:bool)
            n1546 = Not(x=w1999) -> (.not. x?=w2007:bool)
          }
          frame "二维码" {
            w2016 = 2
            w2009 = FALSE ("1 6")
            n1547 = property on="项目信息 2" class="Tbl (严格)"("Disabled"=w2016) -> ()  [unwired: 2 in, 2 out]
            n1548 = property on="加热控制参数" class="Clust (严格)"("Disabled"=w2016) -> ()  [unwired: 2 in, 2 out]
            n1549 = property on="从板号" class="DigNum (严格)"("NumText.BGColor"=u32 6618880) -> ()  [unwired: 2 in, 2 out]
            n1550 = global read "功能码全局.vi" "16"() -> (w2013:bool[])
            n1551 = Index Array(array=w2013, index #1=4 ("索引"), index #2=6 ("索引")) -> (element #1=w2014:bool, element #2=w2011:bool)
            n1552 = Not(x=w2009) -> (.not. x?=w2017:bool)
          }
          frame "从板信息" {
            w2019 = FALSE ("1 6")
            n1553 = Select(t=0, s=w2024, f=1) -> (s? t:f=w2023:i32)
            n1554 = property on="从板号" class="DigNum (严格)"("NumText.BGColor"=u32 16777215) -> ()  [unwired: 2 in, 2 out]
            n1555 = property on="项目信息 2" class="Tbl (严格)"("Disabled"=w2023) -> ()  [unwired: 2 in, 2 out]
            n1556 = property on="加热控制参数" class="Clust (严格)"("Disabled"=w2023) -> ()  [unwired: 2 in, 2 out]
            n1557 = Not(x=w2019) -> (.not. x?=w2027:bool)
            n1558 = local read "从板项目信息"() -> (w2021:bool)
            n1559 = Not(x=w2021) -> (.not. x?=w2020:bool)
          }
          frame "风机关闭温差", "风机关闭温度", "风机开启温差", "风机开启温度", "加热关闭温差", "加热关闭温度", "加热开启温度", "加热控制参数" {
            w2029 = FALSE ("1 6")
            n1560 = property on="从板号" class="DigNum (严格)"("NumText.BGColor"=u32 16777215) -> ()  [unwired: 2 in, 2 out]
            n1561 = Select(t=0, s=w2032, f=1) -> (s? t:f=w2031:i32)
            n1562 = property on="项目信息 2" class="Tbl (严格)"("Disabled"=2) -> ()  [unwired: 2 in, 2 out]
            n1563 = property on="加热控制参数" class="Clust (严格)"("Disabled"=w2031) -> ()  [unwired: 2 in, 2 out]
            n1564 = global read "功能码全局.vi" "16"() -> (w2038:bool[])
            n1565 = Index Array(array=w2038, index #1=5 ("索引"), index #2=7 ("索引")) -> (element #1=w2036:bool, element #2=w2035:bool)
            n1566 = Not(x=w2029) -> (.not. x?=w2041:bool)
          }
          frame "电压个数" {
            w2043 = FALSE ("1 6")
            n1567 = property on="从板号" class="DigNum (严格)"("NumText.BGColor"=u32 16777215) -> ()  [unwired: 2 in, 2 out]
            n1568 = control-ref of="项目信息 2"() -> (w2054:refnum<vi>)
            n1569 = stacked-sequence {
              tunnel: w2054 -> [w2061 w2063 w2072]
              frame #0 {
                n1570 = Bundle(0, 0) -> (w2060:cluster{i32, i32})  [unwired: 1 out]
                n1571 = property class="Tbl (严格)"(reference=w2061, "Index Values"=w2060) -> ()  [unwired: 1 in, 2 out]
              }
              frame #1 {
                n1572 = for {
                  N: 40 -> [_]
                  tunnel: w2063 -> [w2070]
                  i -> [w2065]
                  n1573 = Compound Arithmetic op=ADD(0 ("值"), w2065) -> (w2067:i32)
                  n1574 = Bundle(w2067, 0) -> (w2069:cluster{i32, i32})  [unwired: 1 out]
                  n1575 = property class="Tbl (严格)"(reference=w2070, "Active Cell"=w2069, "Cell BG Color"=u32 16448250) -> ()  [unwired: 1 in, 2 out]
                }
              }
              frame #2 {
                n1576 = for {
                  N: 1 -> [_]
                  tunnel: w2072 -> [w2077]
                  i -> [w2073]
                  n1577 = Bundle(w2073, 0) -> (w2076:cluster{i32, i32})  [unwired: 1 out]
                  n1578 = property class="Tbl (严格)"(reference=w2077, "Active Cell"=w2076, "Cell BG Color"=u32 6618880) -> ()  [unwired: 1 in, 2 out]
                }
              }
            }
            n1579 = Select(t=0, s=w2046, f=1) -> (s? t:f=w2045:i32)
            n1580 = property on="项目信息 2" class="Tbl (严格)"("Disabled"=w2045) -> ()  [unwired: 2 in, 2 out]
            n1581 = property on="加热控制参数" class="Clust (严格)"("Disabled"=2) -> ()  [unwired: 2 in, 2 out]
            n1582 = global read "功能码全局.vi" "15"() -> (w2052:bool[])
            n1583 = Index Array(array=w2052, index #1=0 ("索引"), index #2=4 ("索引")) -> (element #1=w2050:bool, element #2=w2049:bool)
            n1584 = Not(x=w2043) -> (.not. x?=w2056:bool)
          }
          frame "通道电压节数" {
            w2078 = FALSE ("1 6")
            n1585 = property on="从板号" class="DigNum (严格)"("NumText.BGColor"=u32 16777215) -> ()  [unwired: 2 in, 2 out]
            n1586 = control-ref of="项目信息 2"() -> (w2089:refnum<vi>)
            n1587 = stacked-sequence {
              tunnel: w2089 -> [w2096 w2098 w2107]
              frame #0 {
                n1588 = Bundle(22, 0) -> (w2095:cluster{i32, i32})  [unwired: 1 out]
                n1589 = property class="Tbl (严格)"(reference=w2096, "Index Values"=w2095) -> ()  [unwired: 1 in, 2 out]
              }
              frame #1 {
                n1590 = for {
                  N: 40 -> [_]
                  tunnel: w2098 -> [w2105]
                  i -> [w2100]
                  n1591 = Compound Arithmetic op=ADD(0 ("值"), w2100) -> (w2102:i32)
                  n1592 = Bundle(w2102, 0) -> (w2104:cluster{i32, i32})  [unwired: 1 out]
                  n1593 = property class="Tbl (严格)"(reference=w2105, "Active Cell"=w2104, "Cell BG Color"=u32 16448250) -> ()  [unwired: 1 in, 2 out]
                }
              }
              frame #2 {
                n1594 = for {
                  N: 5 -> [_]
                  tunnel: w2107 -> [w2114]
                  i -> [w2110]
                  n1595 = Add(x=22, y=w2110) -> (x+y=w2109:i32)
                  n1596 = Bundle(w2109, 0) -> (w2113:cluster{i32, i32})  [unwired: 1 out]
                  n1597 = property class="Tbl (严格)"(reference=w2114, "Active Cell"=w2113, "Cell BG Color"=u32 6618880) -> ()  [unwired: 1 in, 2 out]
                }
              }
            }
            n1598 = Select(t=0, s=w2081, f=1) -> (s? t:f=w2080:i32)
            n1599 = property on="项目信息 2" class="Tbl (严格)"("Disabled"=w2080) -> ()  [unwired: 2 in, 2 out]
            n1600 = property on="加热控制参数" class="Clust (严格)"("Disabled"=2) -> ()  [unwired: 2 in, 2 out]
            n1601 = global read "功能码全局.vi" "15"() -> (w2087:bool[])
            n1602 = Index Array(array=w2087, index #1=1 ("索引"), index #2=5 ("索引")) -> (element #1=w2085:bool, element #2=w2084:bool)
            n1603 = Not(x=w2078) -> (.not. x?=w2091:bool)
          }
          frame "保险位置" {
            w2115 = FALSE ("1 6")
            n1604 = control-ref of="项目信息 2"() -> (w2126:refnum<vi>)
            n1605 = stacked-sequence {
              tunnel: w2126 -> [w2133 w2135 w2144]
              frame #0 {
                n1606 = Bundle(0, 0) -> (w2132:cluster{i32, i32})  [unwired: 1 out]
                n1607 = property class="Tbl (严格)"(reference=w2133, "Index Values"=w2132) -> ()  [unwired: 1 in, 2 out]
              }
              frame #1 {
                n1608 = for {
                  N: 40 -> [_]
                  tunnel: w2135 -> [w2142]
                  i -> [w2138]
                  n1609 = Add(x=2, y=w2138) -> (x+y=w2137:i32)
                  n1610 = Bundle(w2137, 0) -> (w2141:cluster{i32, i32})  [unwired: 1 out]
                  n1611 = property class="Tbl (严格)"(reference=w2142, "Active Cell"=w2141, "Cell BG Color"=u32 16448250) -> ()  [unwired: 1 in, 2 out]
                }
              }
              frame #2 {
                n1612 = for {
                  N: 20 -> [_]
                  tunnel: w2144 -> [w2151]
                  i -> [w2147]
                  n1613 = Add(x=2, y=w2147) -> (x+y=w2146:i32)
                  n1614 = Bundle(w2146, 0) -> (w2150:cluster{i32, i32})  [unwired: 1 out]
                  n1615 = property class="Tbl (严格)"(reference=w2151, "Active Cell"=w2150, "Cell BG Color"=u32 6618880) -> ()  [unwired: 1 in, 2 out]
                }
              }
            }
            n1616 = property on="从板号" class="DigNum (严格)"("NumText.BGColor"=u32 16777215) -> ()  [unwired: 2 in, 2 out]
            n1617 = Select(t=0, s=w2118, f=1) -> (s? t:f=w2117:i32)
            n1618 = property on="项目信息 2" class="Tbl (严格)"("Disabled"=w2117) -> ()  [unwired: 2 in, 2 out]
            n1619 = property on="加热控制参数" class="Clust (严格)"("Disabled"=2) -> ()  [unwired: 2 in, 2 out]
            n1620 = global read "功能码全局.vi" "15"() -> (w2124:bool[])
            n1621 = Index Array(array=w2124, index #1=2 ("索引"), index #2=6 ("索引")) -> (element #1=w2122:bool, element #2=w2121:bool)
            n1622 = Not(x=w2115) -> (.not. x?=w2128:bool)
          }
          frame "温度个数" {
            w2152 = FALSE ("1 6")
            n1623 = control-ref of="项目信息 2"() -> (w2163:refnum<vi>)
            n1624 = stacked-sequence {
              tunnel: w2163 -> [w2170 w2171 w2181]
              frame #0 {
                n1625 = Bundle(0, 0) -> (w2169:cluster{i32, i32})  [unwired: 1 out]
                n1626 = property class="Tbl (严格)"(reference=w2170, "Index Values"=w2169) -> ()  [unwired: 1 in, 2 out]
              }
              frame #1 {
                n1627 = for {
                  N: 40 -> [_]
                  tunnel: w2171 -> [w2179]
                  i -> [w2174]
                  n1628 = Compound Arithmetic op=ADD(0 ("值"), w2174) -> (w2176:i32)
                  n1629 = Bundle(w2176, 0) -> (w2178:cluster{i32, i32})  [unwired: 1 out]
                  n1630 = property class="Tbl (严格)"(reference=w2179, "Active Cell"=w2178, "Cell BG Color"=u32 16448250) -> ()  [unwired: 1 in, 2 out]
                }
              }
              frame #2 {
                n1631 = for {
                  N: 1 -> [_]
                  tunnel: w2181 -> [w2188]
                  i -> [w2184]
                  n1632 = Add(x=1, y=w2184) -> (x+y=w2183:i32)
                  n1633 = Bundle(w2183, 0) -> (w2187:cluster{i32, i32})  [unwired: 1 out]
                  n1634 = property class="Tbl (严格)"(reference=w2188, "Active Cell"=w2187, "Cell BG Color"=u32 6618880) -> ()  [unwired: 1 in, 2 out]
                }
              }
            }
            n1635 = Select(t=0, s=w2155, f=1) -> (s? t:f=w2154:i32)
            n1636 = property on="项目信息 2" class="Tbl (严格)"("Disabled"=w2154) -> ()  [unwired: 2 in, 2 out]
            n1637 = property on="加热控制参数" class="Clust (严格)"("Disabled"=2) -> ()  [unwired: 2 in, 2 out]
            n1638 = property on="从板号" class="DigNum (严格)"("NumText.BGColor"=u32 16777215) -> ()  [unwired: 2 in, 2 out]
            n1639 = global read "功能码全局.vi" "15"() -> (w2161:bool[])
            n1640 = Index Array(array=w2161, index #1=3 ("索引"), index #2=7 ("索引")) -> (element #1=w2159:bool, element #2=w2158:bool)
            n1641 = Not(x=w2152) -> (.not. x?=w2165:bool)
          }
          frame "SOC过低", "电压不均衡", "电压过低", "电压过高", "温度不均衡", "温度过低", "温度过高", "一级故障阀值" {
            w2189 = FALSE ("1 6")
            n1642 = property on="从板号" class="DigNum (严格)"("NumText.BGColor"=u32 16777215) -> ()  [unwired: 2 in, 2 out]
            n1643 = Select(t=0, s=w2191, f=1) -> (s? t:f=w2192:i32)
            n1644 = property on="一级故障 6" class="Clust (严格)"("DisabledEnum"=w2192) -> ()  [unwired: 2 in, 2 out]
            n1645 = global read "功能码全局.vi" "18"() -> (w2198:bool[])
            n1646 = Index Array(array=w2198, index #1=2 ("索引"), index #2=5 ("索引")) -> (element #1=w2196:bool, element #2=w2195:bool)
            n1647 = Not(x=w2189) -> (.not. x?=w2200:bool)
          }
          frame "SOC过低(2)", "电压不均衡(2)", "电压过低(2)", "电压过高(2)", "二级故障阀值", "温度不均衡(2)", "温度过低(2)", "温度过高(2)" {
            w2202 = FALSE ("1 6")
            n1648 = property on="从板号" class="DigNum (严格)"("NumText.BGColor"=u32 16777215) -> ()  [unwired: 2 in, 2 out]
            n1649 = Select(t=0, s=w2205, f=1) -> (s? t:f=w2204:i32)
            n1650 = property on="一级故障 7" class="Clust (严格)"("DisabledEnum"=w2204) -> ()  [unwired: 2 in, 2 out]
            n1651 = global read "功能码全局.vi" "18"() -> (w2211:bool[])
            n1652 = Index Array(array=w2211, index #1=3 ("索引"), index #2=6 ("索引")) -> (element #1=w2209:bool, element #2=w2208:bool)
            n1653 = Not(x=w2202) -> (.not. x?=w2213:bool)
          }
          frame "SOC过低(3)", "电压不均衡(3)", "电压过低(3)", "电压过高(3)", "三级故障阀值", "温度不均衡(3)", "温度过低(3)", "温度过高(3)" {
            w2215 = FALSE ("1 6")
            n1654 = property on="从板号" class="DigNum (严格)"("NumText.BGColor"=u32 16777215) -> ()  [unwired: 2 in, 2 out]
            n1655 = Select(t=0, s=w2218, f=1) -> (s? t:f=w2217:i32)
            n1656 = property on="一级故障 8" class="Clust (严格)"("DisabledEnum"=w2217) -> ()  [unwired: 2 in, 2 out]
            n1657 = global read "功能码全局.vi" "18"() -> (w2224:bool[])
            n1658 = Index Array(array=w2224, index #1=4 ("索引"), index #2=7 ("索引")) -> (element #1=w2222:bool, element #2=w2221:bool)
            n1659 = Not(x=w2215) -> (.not. x?=w2226:bool)
          }
          frame "快换参数" {
            w2228 = FALSE ("1 6")
            n1660 = Select(t=0, s=w2249, f=1) -> (s? t:f=w2248:i32)
            n1661 = property on="电池组信息" class="Clust (严格)"("Disabled"=w2248) -> ()  [unwired: 2 in, 2 out]
            n1662 = property on="从板号" class="DigNum (严格)"("NumText.BGColor"=u32 16777215) -> ()  [unwired: 2 in, 2 out]
            n1663 = global read "功能码全局.vi" "24"() -> (w2245:bool[])
            n1664 = global read "功能码全局.vi" "23"() -> (w2246:bool[])
            n1665 = Index Array(array=w2245) -> (element #3=w2235:bool, element #4=w2234:bool, element #5=w2233:bool, element #6=w2232:bool, element #7=w2231:bool, element #8=w2230:bool)  [unwired: 8 in, 2 out]
            n1666 = Index Array(array=w2246) -> (element #3=w2244:bool, element #4=w2243:bool, element #5=w2242:bool, element #6=w2241:bool, element #7=w2240:bool, element #8=w2239:bool)  [unwired: 8 in, 2 out]
            n1667 = Build Array(w2235, w2234, w2233, w2232, w2231, w2230) -> (w2236:bool[])
            n1668 = Build Array(w2244, w2243, w2242, w2241, w2240, w2239) -> (w2238:bool[])
            n1669 = And Array Elements(Boolean array=w2236) -> (logical AND=w2229:bool)
            n1670 = And Array Elements(Boolean array=w2238) -> (logical AND=w2237:bool)
            n1671 = Not(x=w2228) -> (.not. x?=w2252:bool)
          }
          frame "电池包信息1" {
            w2257 = 2
            w2265 = 2
            w2256 = 2
            w2254 = FALSE ("1 6")
            n1672 = Select(t=0, s=w2262, f=1) -> (s? t:f=w2255:i32)
            n1673 = property on="串联数" class="DigNum (严格)"("Disabled"=w2255) -> ()  [unwired: 2 in, 2 out]
            n1674 = property on="并联数" class="DigNum (严格)"("Disabled"=w2255) -> ()  [unwired: 2 in, 2 out]
            n1675 = property on="电池厂家" class="DigNum (严格)"("Disabled"=w2255) -> ()  [unwired: 2 in, 2 out]
            n1676 = property on="电池类型" class="DigNum (严格)"("Disabled"=w2255) -> ()  [unwired: 2 in, 2 out]
            n1677 = property on="额定能量" class="DigNum (严格)"("Disabled"=w2255) -> ()  [unwired: 2 in, 2 out]
            n1678 = property on="额定容量" class="DigNum (严格)"("Disabled"=w2255) -> ()  [unwired: 2 in, 2 out]
            n1679 = property on="实际容量" class="DigNum (严格)"("Disabled"=w2255) -> ()  [unwired: 2 in, 2 out]
            n1680 = property on="电池组信息" class="Clust (严格)"("Disabled"=w2255) -> ()  [unwired: 2 in, 2 out]
            n1681 = property on="生产日期" class="Str"("DisabledEnum"=w2255) -> ()  [unwired: 2 in, 2 out]
            n1682 = property on="车牌号" class="Str"("DisabledEnum"=w2256) -> ()  [unwired: 2 in, 2 out]
            n1683 = property on="产权标识" class="DigNum (严格)"("Disabled"=w2255) -> ()  [unwired: 2 in, 2 out]
            n1684 = property on="应用车型" class="DigNum (严格)"("Disabled"=w2255) -> ()  [unwired: 2 in, 2 out]
            n1685 = property on="额定总压" class="DigNum (严格)"("Disabled"=w2255) -> ()  [unwired: 2 in, 2 out]
            n1686 = property on="电池包序号" class="DigNum (严格)"("DisabledEnum"=w2255) -> ()  [unwired: 2 in, 2 out]
            n1687 = property on="电池包组号" class="DigNum (严格)"("DisabledEnum"=w2256) -> ()  [unwired: 2 in, 2 out]
            n1688 = property on="最大允许单体电压" class="DigNum (严格)"("Disabled"=w2265) -> ()  [unwired: 2 in, 2 out]
            n1689 = property on="最大允许总电压" class="DigNum (严格)"("Disabled"=w2265) -> ()  [unwired: 2 in, 2 out]
            n1690 = property on="最大允许温度" class="DigNum (严格)"("Disabled"=w2265) -> ()  [unwired: 2 in, 2 out]
            n1691 = property on="最小允许温度" class="DigNum (严格)"("Disabled"=w2265) -> ()  [unwired: 2 in, 2 out]
            n1692 = property on="最大允许充电电流" class="DigNum (严格)"("Disabled"=w2265) -> ()  [unwired: 2 in, 2 out]
            n1693 = property on="最小允许充电电流" class="DigNum (严格)"("Disabled"=w2265) -> ()  [unwired: 2 in, 2 out]
            n1694 = property on="最小允许单体电压" class="DigNum (严格)"("Disabled"=w2265) -> ()  [unwired: 2 in, 2 out]
            n1695 = property on="电流步长" class="DigNum (严格)"("Disabled"=w2265) -> ()  [unwired: 2 in, 2 out]
            n1696 = property on="SOC" class="DigNum (严格)"("Disabled"=w2265) -> ()  [unwired: 2 in, 2 out]
            n1697 = property on="充电总安时" class="DigNum (严格)"("Disabled"=w2265) -> ()  [unwired: 2 in, 2 out]
            n1698 = property on="放电总安时" class="DigNum (严格)"("Disabled"=w2265) -> ()  [unwired: 2 in, 2 out]
            n1699 = property on="放空次数" class="DigNum (严格)"("DisabledEnum"=w2257) -> ()  [unwired: 2 in, 2 out]
            n1700 = property on="充满次数" class="DigNum (严格)"("DisabledEnum"=w2257) -> ()  [unwired: 2 in, 2 out]
            n1701 = property on="充电次数" class="DigNum (严格)"("DisabledEnum"=w2257) -> ()  [unwired: 2 in, 2 out]
            n1702 = global read "功能码全局.vi" "24"() -> (w2260:bool[])
            n1703 = global read "功能码全局.vi" "23"() -> (w2261:bool[])
            n1704 = Index Array(array=w2260) -> (element #3=w2258:bool)  [unwired: 8 in, 7 out]
            n1705 = Index Array(array=w2261) -> (element #3=w2259:bool)  [unwired: 8 in, 7 out]
            n1706 = Not(x=w2254) -> (.not. x?=w2266:bool)
          }
          frame "电池包组号" {
            w2271 = 2
            w2270 = 2
            w2280 = 2
            w2272 = 2
            w2281 = 2
            w2268 = FALSE ("1 6")
            n1707 = property on="串联数" class="DigNum (严格)"("Disabled"=w2281) -> ()  [unwired: 2 in, 2 out]
            n1708 = property on="并联数" class="DigNum (严格)"("Disabled"=w2281) -> ()  [unwired: 2 in, 2 out]
            n1709 = property on="电池厂家" class="DigNum (严格)"("Disabled"=w2281) -> ()  [unwired: 2 in, 2 out]
            n1710 = property on="电池类型" class="DigNum (严格)"("Disabled"=w2281) -> ()  [unwired: 2 in, 2 out]
            n1711 = property on="额定能量" class="DigNum (严格)"("Disabled"=w2281) -> ()  [unwired: 2 in, 2 out]
            n1712 = property on="额定容量" class="DigNum (严格)"("Disabled"=w2281) -> ()  [unwired: 2 in, 2 out]
            n1713 = property on="实际容量" class="DigNum (严格)"("Disabled"=w2281) -> ()  [unwired: 2 in, 2 out]
            n1714 = Select(t=0, s=w2277, f=1) -> (s? t:f=w2269:i32)
            n1715 = property on="生产日期" class="Str"("DisabledEnum"=w2271) -> ()  [unwired: 2 in, 2 out]
            n1716 = property on="电池包序号" class="DigNum (严格)"("DisabledEnum"=w2271) -> ()  [unwired: 2 in, 2 out]
            n1717 = property on="车牌号" class="Str"("DisabledEnum"=w2271) -> ()  [unwired: 2 in, 2 out]
            n1718 = property on="电池包组号" class="DigNum (严格)"("DisabledEnum"=w2269) -> ()  [unwired: 2 in, 2 out]
            n1719 = property on="电池组信息" class="Clust (严格)"("Disabled"=w2269) -> ()  [unwired: 2 in, 2 out]
            n1720 = property on="产权标识" class="DigNum (严格)"("Disabled"=w2272) -> ()  [unwired: 2 in, 2 out]
            n1721 = property on="应用车型" class="DigNum (严格)"("Disabled"=w2272) -> ()  [unwired: 2 in, 2 out]
            n1722 = property on="额定总压" class="DigNum (严格)"("Disabled"=w2272) -> ()  [unwired: 2 in, 2 out]
            n1723 = property on="放空次数" class="DigNum (严格)"("DisabledEnum"=w2270) -> ()  [unwired: 2 in, 2 out]
            n1724 = property on="充满次数" class="DigNum (严格)"("DisabledEnum"=w2270) -> ()  [unwired: 2 in, 2 out]
            n1725 = property on="充电次数" class="DigNum (严格)"("DisabledEnum"=w2270) -> ()  [unwired: 2 in, 2 out]
            n1726 = property on="最大允许单体电压" class="DigNum (严格)"("Disabled"=w2280) -> ()  [unwired: 2 in, 2 out]
            n1727 = property on="最大允许总电压" class="DigNum (严格)"("Disabled"=w2280) -> ()  [unwired: 2 in, 2 out]
            n1728 = property on="最大允许温度" class="DigNum (严格)"("Disabled"=w2280) -> ()  [unwired: 2 in, 2 out]
            n1729 = property on="最小允许温度" class="DigNum (严格)"("Disabled"=w2280) -> ()  [unwired: 2 in, 2 out]
            n1730 = property on="最大允许充电电流" class="DigNum (严格)"("Disabled"=w2280) -> ()  [unwired: 2 in, 2 out]
            n1731 = property on="最小允许充电电流" class="DigNum (严格)"("Disabled"=w2280) -> ()  [unwired: 2 in, 2 out]
            n1732 = property on="最小允许单体电压" class="DigNum (严格)"("Disabled"=w2280) -> ()  [unwired: 2 in, 2 out]
            n1733 = property on="电流步长" class="DigNum (严格)"("Disabled"=w2280) -> ()  [unwired: 2 in, 2 out]
            n1734 = property on="SOC" class="DigNum (严格)"("Disabled"=w2280) -> ()  [unwired: 2 in, 2 out]
            n1735 = property on="充电总安时" class="DigNum (严格)"("Disabled"=w2280) -> ()  [unwired: 2 in, 2 out]
            n1736 = property on="放电总安时" class="DigNum (严格)"("Disabled"=w2280) -> ()  [unwired: 2 in, 2 out]
            n1737 = global read "功能码全局.vi" "24"() -> (w2275:bool[])
            n1738 = global read "功能码全局.vi" "23"() -> (w2276:bool[])
            n1739 = Index Array(array=w2275) -> (element #3=w2273:bool)  [unwired: 8 in, 7 out]
            n1740 = Index Array(array=w2276) -> (element #3=w2274:bool)  [unwired: 8 in, 7 out]
            n1741 = Not(x=w2268) -> (.not. x?=w2282:bool)
          }
          frame "充放电安时" {
            w2286 = 2
            w2285 = 2
            w2295 = 2
            w2296 = 2
            w2298 = 2
            w2284 = FALSE ("1 6")
            n1742 = property on="串联数" class="DigNum (严格)"("Disabled"=w2298) -> ()  [unwired: 2 in, 2 out]
            n1743 = property on="并联数" class="DigNum (严格)"("Disabled"=w2298) -> ()  [unwired: 2 in, 2 out]
            n1744 = property on="电池厂家" class="DigNum (严格)"("Disabled"=w2298) -> ()  [unwired: 2 in, 2 out]
            n1745 = property on="电池类型" class="DigNum (严格)"("Disabled"=w2298) -> ()  [unwired: 2 in, 2 out]
            n1746 = property on="额定能量" class="DigNum (严格)"("Disabled"=w2298) -> ()  [unwired: 2 in, 2 out]
            n1747 = property on="额定容量" class="DigNum (严格)"("Disabled"=w2298) -> ()  [unwired: 2 in, 2 out]
            n1748 = property on="实际容量" class="DigNum (严格)"("Disabled"=w2298) -> ()  [unwired: 2 in, 2 out]
            n1749 = Select(t=0, s=w2292, f=1) -> (s? t:f=w2291:i32)
            n1750 = property on="生产日期" class="Str"("DisabledEnum"=w2286) -> ()  [unwired: 2 in, 2 out]
            n1751 = property on="电池包序号" class="DigNum (严格)"("DisabledEnum"=w2286) -> ()  [unwired: 2 in, 2 out]
            n1752 = property on="车牌号" class="Str"("DisabledEnum"=w2286) -> ()  [unwired: 2 in, 2 out]
            n1753 = property on="电池包组号" class="DigNum (严格)"("DisabledEnum"=w2286) -> ()  [unwired: 2 in, 2 out]
            n1754 = property on="电池组信息" class="Clust (严格)"("Disabled"=w2291) -> ()  [unwired: 2 in, 2 out]
            n1755 = property on="额定总压" class="DigNum (严格)"("Disabled"=2) -> ()  [unwired: 2 in, 2 out]
            n1756 = property on="产权标识" class="DigNum (严格)"("Disabled"=w2296) -> ()  [unwired: 2 in, 2 out]
            n1757 = property on="应用车型" class="DigNum (严格)"("Disabled"=w2296) -> ()  [unwired: 2 in, 2 out]
            n1758 = property on="放空次数" class="DigNum (严格)"("DisabledEnum"=w2285) -> ()  [unwired: 2 in, 2 out]
            n1759 = property on="充满次数" class="DigNum (严格)"("DisabledEnum"=w2285) -> ()  [unwired: 2 in, 2 out]
            n1760 = property on="充电次数" class="DigNum (严格)"("DisabledEnum"=w2285) -> ()  [unwired: 2 in, 2 out]
            n1761 = property on="最大允许单体电压" class="DigNum (严格)"("Disabled"=w2295) -> ()  [unwired: 2 in, 2 out]
            n1762 = property on="最大允许总电压" class="DigNum (严格)"("Disabled"=w2295) -> ()  [unwired: 2 in, 2 out]
            n1763 = property on="最大允许温度" class="DigNum (严格)"("Disabled"=w2295) -> ()  [unwired: 2 in, 2 out]
            n1764 = property on="最小允许温度" class="DigNum (严格)"("Disabled"=w2295) -> ()  [unwired: 2 in, 2 out]
            n1765 = property on="最大允许充电电流" class="DigNum (严格)"("Disabled"=w2295) -> ()  [unwired: 2 in, 2 out]
            n1766 = property on="最小允许充电电流" class="DigNum (严格)"("Disabled"=w2295) -> ()  [unwired: 2 in, 2 out]
